vi "SubVI_CreateDecoder.vi"(0 "pixelFormat":string, 1 "redGain":dbl, 2 "greenGain":dbl, 3 "blueGain":dbl, 5 "height":u32, 7 "width":u32, 9 "Output Bitdepth":u16(ring)=32 items=["RGB32"=32, "RGB64"=64], 11 "error in":errorcluster, 12 "Bayer Decode Algorithm":T1, 13 "Right Shift Data?":bool, 14 "needsSwap":bool) -> (8 "decoder":u64, 15 "error":errorcluster)   [LabVIEW 2021]
uses:
  bayer_decode.ctl
  niimaqdx.dll
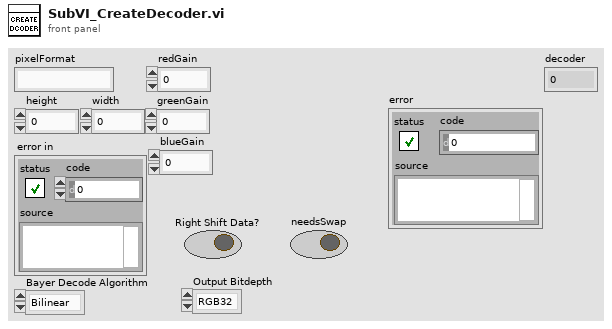
[diagram p1: front panel]
types:
  T1 = typedef "bayer_decode.ctl" = enum16{"Bilinear", "VNG"}
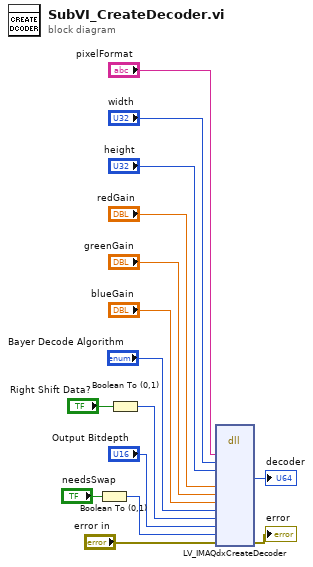
[diagram p0: block diagram]
diagram:
  n1 = Boolean To (0,1)(Boolean="needsSwap") -> (0, 1=w1:i16)
  n2 = Boolean To (0,1)(Boolean="Right Shift Data?") -> (0, 1=w3:i16)
  n3 = dll-call lib="niimaqdx.dll" fn="LV_IMAQdxCreateDecoder"("pixelFormat"="pixelFormat", "width"="width", "height"="height", "redGain"="redGain", "greenGain"="greenGain", "blueGain"="blueGain", "decodeMethod"="Bayer Decode Algorithm", "rightShift"=w3, "outputDepth"="Output Bitdepth", "needSwap"=w1, "error"="error in") -> ("decoderRef"=→"decoder":u64, "error"=→"error":errorcluster)  [unwired: 3 in, 14 out]
